vi "菜单-执行.vi"(8 "error in (no error)":errorcluster caption="错误输入（无错误）", 11 "程序响应 输入":refnum<class "程序响应.lvclass">) -> (0 "error out":errorcluster caption="错误输出", 3 "程序响应 输出":refnum<class "程序响应.lvclass">)   [LabVIEW 2018, in "程序响应.lvlib" / "程序响应.lvclass"]
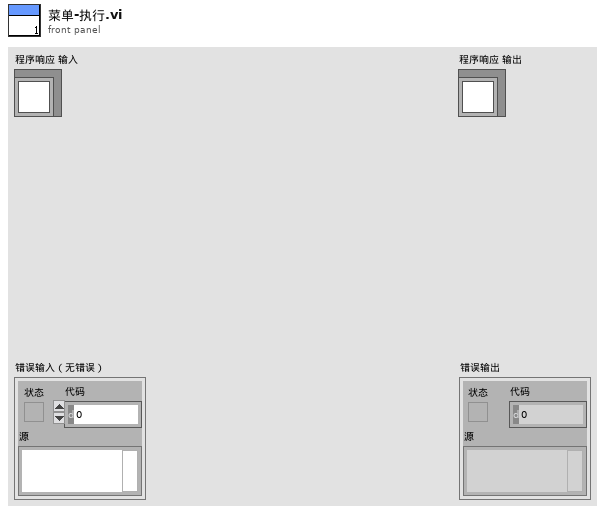
[diagram p1: front panel]
types:
  T1 = enum16{"open", "replace", "create", "open or create", "replace or create", "replace or create with confirmation"}
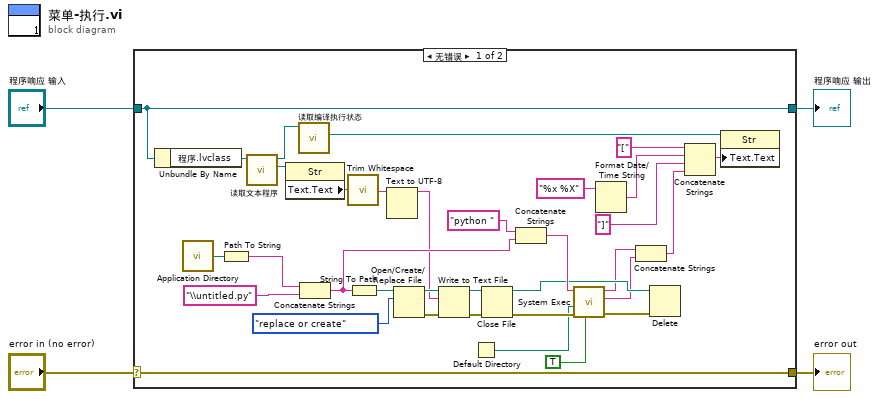
[diagram p0: block diagram]
diagram:
  n1 = case shown="无错误" "error in (no error)" {
    selector: "error in (no error)" -> [w38 w40]
    tunnel: [w38 w40] -> w3
    tunnel: [w37 w39] -> w1
    tunnel: "程序响应 输入" -> [w37 w39]
    frame No Error {
      n2 = Unbundle By Name(w37) -> ("程序.lvclass"=w36:refnum<class "程序.lvclass">)
      n3 = call <vilib>:"Application Directory.vi"() -> ("Application Directory"=w33:path)
      n4 = Path To String(path=w33) -> (string=w32:string)
      n5 = call-dynamic "读取文本程序.vi"("程序输入"=w36) -> ("文本程序"=w35:refnum<vi>, "程序输出"=w14:refnum<class "程序.lvclass">)  [unwired: 8 in, 1 out]
      n6 = property class="Str"(reference=w35) -> ("Text.Text"=w34:string)  [unwired: 1 in, 2 out]
      n7 = call-dynamic "读取编译执行状态.vi"("程序输入"=w14) -> ("编译执行状态"=w13:refnum<vi>)  [unwired: 8 in, 2 out]
      n8 = Concatenate Strings(w32, "\\untitled.py" ("字符串")) -> (w23:string)
      n9 = call <vilib>:"Trim Whitespace.vi"("string"=w34) -> ("trimmed string"=w6:string)  [unwired: 1 in]
      n10 = String To Path(string=w23) -> (path=w30:path)
      n11 = Text to UTF-8(11:w6) -> (3:w5:string)  [unwired: 2 in, 1 out]
      n12 = Open/Create/Replace File(file path (use dialog)=w30, operation (0:open)=T1."replace or create" ("操作(0:open)")) -> (refnum out=w29:refnum<file>, error out=w28:errorcluster)  [unwired: 4 in, 1 out]
      n13 = Write to Text File(file (use dialog)=w29, text=w5, error in=w28) -> (refnum out=w27:refnum<file>, error out=w26:errorcluster)  [unwired: 1 in, 1 out]
      n14 = Default Directory() -> (w17:path)
      n15 = Close File(refnum=w27, error in=w26) -> (path=w20:path, error out=w24:errorcluster)
      n16 = Concatenate Strings("python " ("字符串"), w23) -> (w22:string)
      n17 = call <vilib>:"System Exec.vi"("run minimized? (F)"=TRUE, "error in (no error)"=w24, "working directory"=w17, "command line"=w22) -> ("error out"=w21:errorcluster, "standard error"=w19:string, "standard output"=w18:string)  [unwired: 4 in, 1 out]
      n18 = Format Date/Time String(time format string (%c)="%x %X" ("时间格式字符串(%c)")) -> (date/time string=w12:string)  [unwired: 2 in]
      n19 = Concatenate Strings(w18, w19) -> (w7:string)
      n20 = Delete(path (use dialog)=w20, error in=w21) -> ()  [unwired: 3 in, 3 out]
      n21 = Concatenate Strings("[" ("字符串"), w12, "]" ("字符串"), w7) -> (w8:string)
      n22 = property class="Str"(reference=w13, "Text.Text"=w8) -> ()  [unwired: 1 in, 2 out]
    }
    frame Error {
    }
  }
  "error out" <- w3
  "程序响应 输出" <- w1
